vi "Convert TDMS File To No DAQmx Raw 2012 NIVerified.vi"(2 "New File":path, 8 "File With Raw DAQmx":path) -> ()   [LabVIEW 2017]
doc: "Open a TDMS file with DQAmxRaw data in it, write all of the data to a new file. The DAQmxRaw datatype is used for high throughput data file writing. Raw ADC Data is stored with scaling factors in the DAQmxRaw datatype. The decoding information for this datatype is not provided by NI in the tdms documentation at: http://zone.ni.com/devzone/cda/tut/p/id/5696. This VI demonstrates how a simple VI can be used to open a TDMS file which contains data in the DAQmxRaw data type and write it to another file (this operation converts the data in the file to the supported data types available to users in the TDMS documentation).\n\nThis will convert DAQmx Raw data which is problematic for reading with other tools (http://www.mathworks.com/matlabcentral/fileexchange/44206-converttdms-v10)."
panel:
  out "Error":errorcluster
  # "Overview: Very simple utility to read in a TDMS file and the write out data to a new TDMS file (which does not use the DAQmx Raw Data type).\nRequirements: LabVIEW 2012 (or compatible)\nInstructions:\n1. Run the VI.\n2. Select File to be converted.\n3. Copy File name from above and change or append to name.\n4. Press OK to convert button."
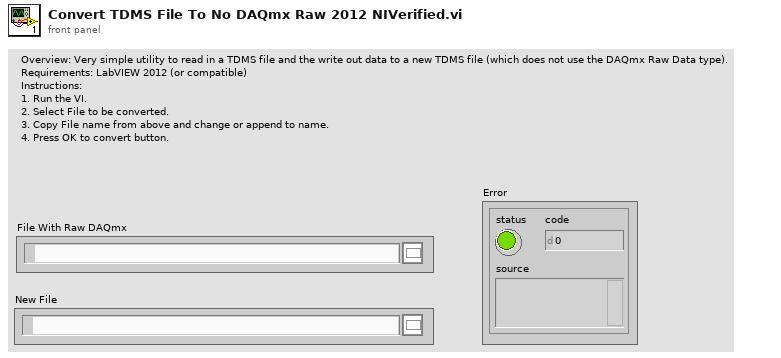
[diagram p1: front panel]
types:
  T1 = enum16{"open", "open or create", "create or replace", "create", "open (read-only)"}
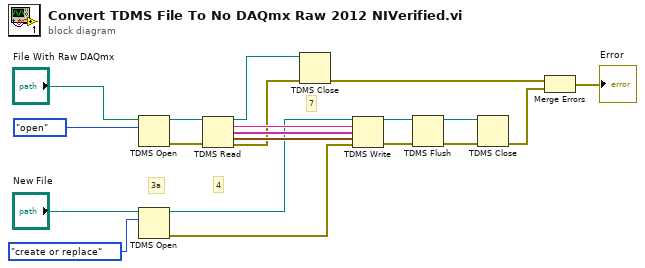
[diagram p0: block diagram]
diagram:
  # "3a"
  # "7"
  # "4"
  n1 = TDMS Open(10:T1."open" ("operation (0:open)"), 11:"File With Raw DAQmx") -> (0:w16:errorcluster, 3:w17:refnum<k34>)  [unwired: 5 in]
  n2 = TDMS Open(10:T1."create or replace" ("operation (0:open)"), 11:"New File") -> (0:w4:errorcluster, 3:w13:refnum<k34>)  [unwired: 5 in]
  n3 = TDMS Read(0:w17, 11:w16) -> (4:w9:refnum<k34>, 6:w20:string, 8:w19:string[], 10:w18:waveform(dbl)[], 15:w10:errorcluster)  [unwired: 6 in, 1 out]
  n4 = TDMS Close(8:w10, 11:w9) -> (0:w3:errorcluster)  [unwired: 1 out]
  n5 = TDMS Write(0:w13, 5:w20, 7:w19, 9:w18, 11:w4) -> (4:w7:refnum<k34>, 15:w8:errorcluster)  [unwired: 1 in, 2 out]
  n6 = TDMS Flush(4:w8, 7:w7) -> (0:w6:errorcluster, 3:w5:refnum<k34>)
  n7 = TDMS Close(8:w6, 11:w5) -> (0:w2:errorcluster)  [unwired: 1 out]
  n8 = Merge Errors(w3, w2) -> (→"Error":errorcluster)
